vi "2D Array to Dynamic Data.vi"(8 "Error In":errorcluster, 10 "Channels":string[](array[string]), 11 "Array":dbl[][](array[numeric])) -> (0 "Error Out":errorcluster, 2 "Channels out":string[](array[string]), 3 "Dynamic Data Type":dynamicdata(graph))   [LabVIEW 2016]
panel:
  out "Array 2":dbl[](array[numeric])
  out "channel number":i32
  out "rows":i32
  in  "file path":path=path "C:/Data/test.tdms"
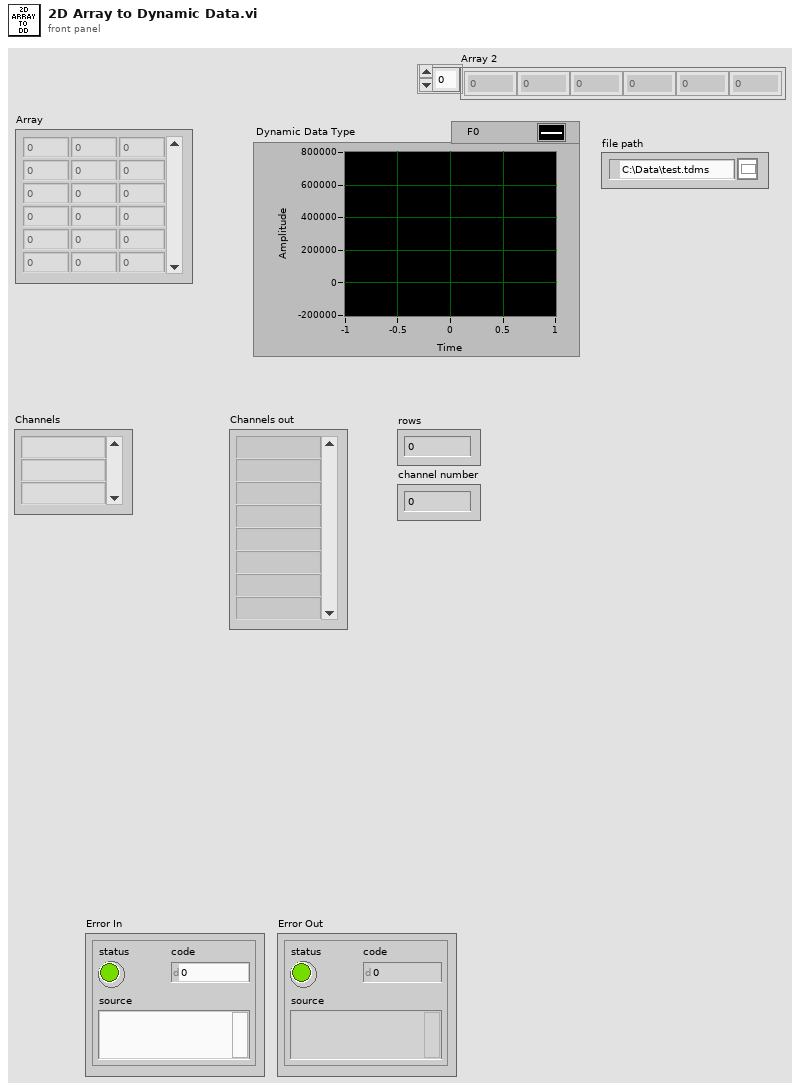
[diagram p1: front panel]
types:
  T1 = enum16{"open", "open or create", "create or replace", "create", "open (read-only)"}
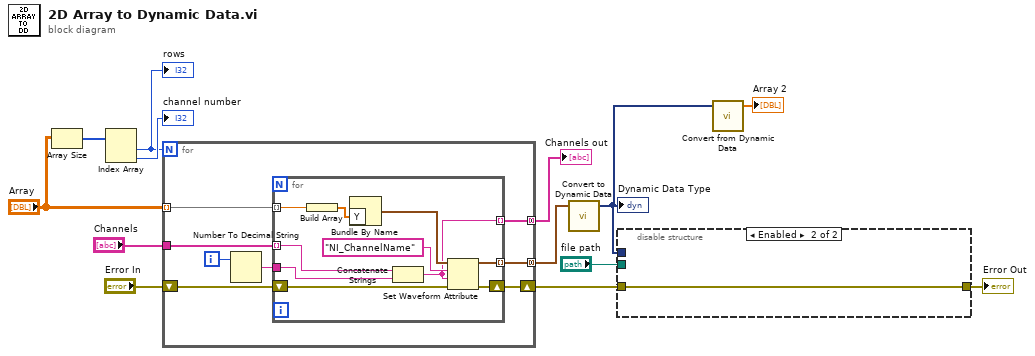
[diagram p0: block diagram]
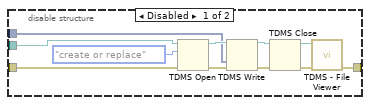
[diagram p2: hidden frame]
diagram:
  n1 = Array Size(array="Array") -> (size(s)=w12:i32[])
  n2 = Index Array(array=w12) -> (element #1=w10:i32, element #2=→"channel number":i32)  [unwired: 2 in]
  "rows" <- w10
  n3 = for {
    N: w10 -> [_]
    tunnel: "Channels" -> [w20]
    tunnel: [w18] -> w9 mode=concatenating
    tunnel: "Array" -> [w17] mode=indexing
    tunnel: [w16] -> w8 mode=concatenating
    shift-right: [w14] -> w7
    shift-left: "Error In" -> [w15]
    i -> [w21]
    n4 = Number To Decimal String(number=w21) -> (decimal integer string=w19:string)  [unwired: 1 in]
    n5 = for {
      tunnel: w20 -> [w31] mode=indexing
      tunnel: w19 -> [w30]
      tunnel: [w22] -> w18 mode=indexing
      tunnel: w17 -> [w29] mode=indexing
      tunnel: [w26] -> w16 mode=indexing
      shift-right: [w24] -> w14
      shift-left: w15 -> [w25]
      n6 = Build Array(w29) -> (w28:dbl[])
      n7 = Bundle By Name("Y"=w28) -> (w27:waveform(dbl))  [unwired: 1 in]
      n8 = Concatenate Strings(w31, w30) -> (w22:string)
      n9 = Set Waveform Attribute(4:w25, 5:w22, 6:"NI_ChannelName" ("name"), 7:w27) -> (0:w24:errorcluster, 3:w26:waveform(dbl))  [unwired: 1 out]
    }
  }
  "Channels out" <- w9
  n10 = call "Convert to Dynamic Data"("Array of Waveforms"=w8) -> ("Dynamic Data Type"=w2:dynamicdata)  [unwired: 3 in]
  "Dynamic Data Type" <- w2
  n11 = disable-structure shown="Enabled" {
    disable-tunnel: "file path" -> [w42 _]
    disable-tunnel: w2 -> [w38 _]
    disable-tunnel: w7 -> [w33 w43]
    disable-tunnel: [w32 w43] -> w3
    frame Disabled {
      n12 = TDMS Open(8:w33, 10:T1."create or replace" ("operation (0:open)"), 11:w42) -> (0:w39:errorcluster, 3:w40:refnum<k34>)  [unwired: 4 in]
      n13 = TDMS Write(0:w40, 9:w38, 11:w39) -> (4:w36:refnum<k34>, 15:w37:errorcluster)  [unwired: 3 in, 2 out]
      n14 = TDMS Close(8:w37, 11:w36) -> (0:w34:errorcluster, 3:w35:path)
      n15 = call <vilib>:"TDMS - File Viewer.vi"("error in (no error)"=w34, "file path"=w35) -> ("error out"=w32:errorcluster)  [unwired: 4 in, 1 out]
    }
    frame Enabled {
    }
  }
  "Error Out" <- w3
  n16 = call "Convert from Dynamic Data"("Dynamic Data Type"=w2) -> ("Array"=→"Array 2":dbl[])  [unwired: 3 in]
